vi "Fast Pixel to Micron.vi"(0 "Refnum In":T2, 11 "error in (no error)":errorcluster, 12 "Conversion Method":u16(ring)=1 items=["Strip Centers", "Signal Fit, Left to Right", "Projection + Signal Fit"]) -> (3 "FFT Angle (Rad)":dbl format="%_6f", 4 "Microns/Pixel":dbl format="%.4f", 6 "Error":dbl format="%.4f", 8 "Corrected":dbl format="%.4f", 10 "Error":dbl format="%.4f", 14 "FFT Error (Rad)":dbl format="%_6f", 15 "error out":errorcluster)   [LabVIEW 2016]
uses:
  <vilib>/Analysis/6fits.llb/Curve Fitting Criteria.ctl
  <vilib>/vision/Image Controls.llb/IMAQ Image.ctl
  <vilib>/measure/mascope.llb/Pulse Measurements 1 chan.vi
  <vilib>/measure/matone.llb/Extract Single Tone Information 1 Chan.vi
  <vilib>/vision/NI_Vision_Development_Module.lvlib
  <vilib>/Analysis/NI_AALBase.lvlib
  <vilib>/measure/NI_MAPro.lvlib
  <vilib>/Analysis/NI_AALPro.lvlib
  <vilib>/Analysis/6fits.llb/Remove Outliers (Range).vi
  <vilib>/Analysis/6fits.llb/Confidence Interval (Linear).vi
panel:
  in  "Tab Control":T1(tab)
  out "Original Image":T2(plugin-control)
  in  "File Path":path=path "D:/Documents/School/Brookhaven/Images/2017-06-15/image_004_600_60_15.png"
  out "Cropped Image":T2(plugin-control)
  in  "Crop Size":i32=1000 min=250 max=2700
  out "Thresholded Image":T2(plugin-control)
  out "FFT Skew Detection":T2(plugin-control)
  in  "Fit Method":T3 items=["Least Square", "Least Absolute Residual", "Bisquare"]
  out "Fit Slopes":dbl[](array[numeric]) format="%^_3e"
  out "Error (Slope)":dbl format="%.5f"
  out "Error (Radians)":dbl format="%.5f"
  out "Radians":dbl format="%.5f"
  out "Slope":dbl format="%.5f"
  in  "Minimum Width":i32=7 min=3 max=15
  in  "Point Constraint (Pixels)":dbl=40.0 min=0.0 max=100.0 step=1.0 format="%#.2f"
  in  "Keep N Devs":dbl=2.0 min=1.0 max=5.0
  in  "Minimum Height":dbl=200.0 min=0.0 max=255.0
  out "Num slope errors":i32
  out "Num slopes":i32
  in  "Use Center Nth of Strips":i32=4 min=1 max=10 step=1
  out "Slope Error":dbl[](array[numeric]) format="%^#_3e"
  out "FFT Angle (Deg)":dbl format="%_6g"
  out "FFT Error (Deg)":dbl format="%_6g"
  out "Distribution of Pitches":T4(graph)
  out "Mean (Pixels)":dbl format="%.4f"
  out "Std. Dev.":dbl format="%.4f"
  out "N":i32
  out "Std. Dev / Sqrt(N)":dbl format="%#.4g"
  in  "Max Value":dbl=70.0 format="%#_13g"
  in  "Min Value":dbl=40.0 min=30.0 max=75.0
  in  "Standard Devs":dbl=3.0 min=0.0 max=5.0
  # "FFT Skew Detection"
  # "Pixel to Micron Conversion"
  # "Histogram"
  # "Absolute Constraint"
  # "Relative Constraint"
  # "Skew Correction (Experimental)"
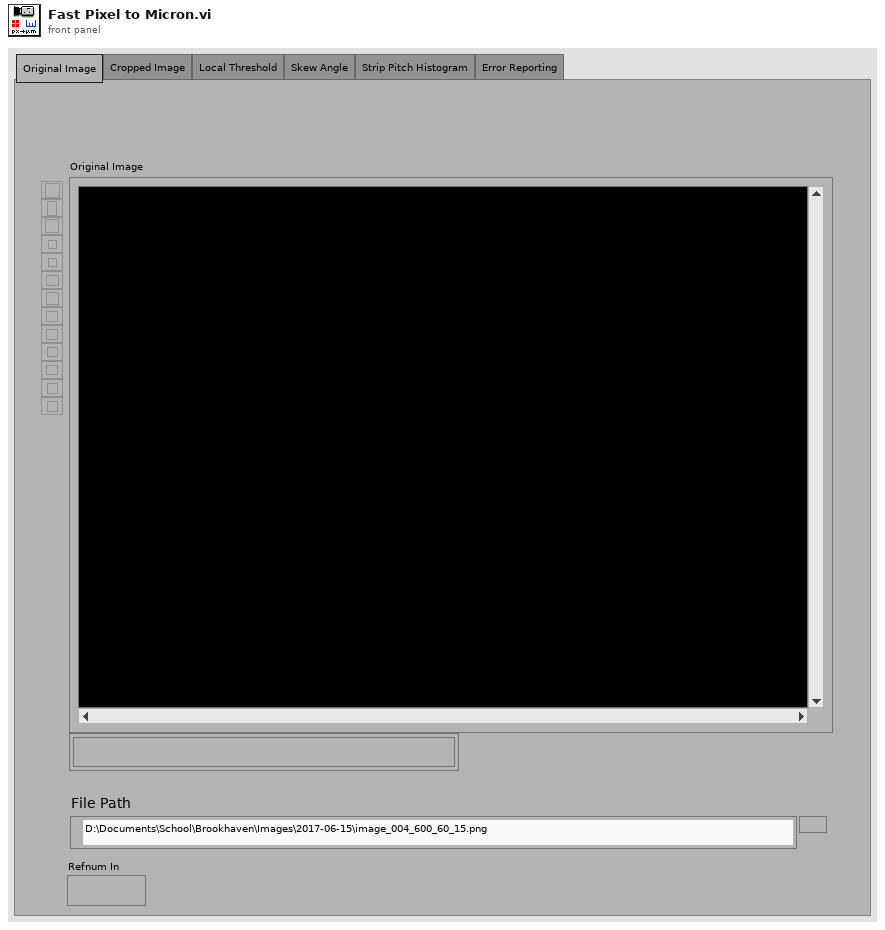
[diagram p1: front panel]
types:
  T1 = enum32{"Original Image", "Cropped Image", "Local Threshold", "Skew Angle", "Strip Pitch Histogram", "Error Reporting"}
  T2 = typedef "IMAQ Image.ctl" = refnum<image>
  T3 = typedef "NI_AALPro.lvlib/Curve Fitting Criteria.ctl" = u16
  T4 = cluster{"X Values":dbl[], "Histogram: h(x)":i32[]}
  T5 = typedef "Image Type" = u32
  T6 = cluster{"high ref level":dbl, "mid ref level":dbl, "low ref level":dbl, "ref units":u16}
  T7 = cluster{"pulse center":dbl, "ref levels":cluster{"high ref level":dbl, "mid ref level":dbl, "low ref level":dbl, "ref units":u16}}
  T8 = cluster{"Numeric":dbl, "Numeric":dbl, "Numeric":dbl}[]
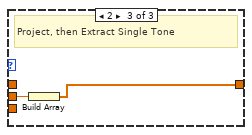
[diagram p10: hidden frame]
diagram:
  n1 = Not A Number/Path/Refnum?(number/path/refnum="Refnum In") -> (NaN/Path/Refnum?=w4:bool)
  n2 = case shown="True" w4 {
    tunnel: [w49 w52] -> w47
    tunnel: [w48 w51] -> w20
    tunnel: "error in (no error)" -> [w48 w50]
    tunnel: "Refnum In" -> [w49 _]
    frame False {
    }
    frame True {
      n3 = in-place {
        in-place-border: [w58] -> w52
        in-place-border: [w55] -> w51
        in-place-border: w50 -> [w54]
        w59 = T5 0 items=["Grayscale (U8)", "Grayscale (I16)", "Grayscale (SGL)", "Complex (CSG)", "RGB (U32)", "HSL (U32)", "RGB (U64)", "Grayscale (U16)"] ("Image Type")
        # "Load test image"
        n4 = call "IMAQ Create"("Image Name"="Test Image", "Image Type"=w59, "error in (no error)"=w54) -> ("New Image"=w60:T2, "error out"=w56:errorcluster)  [unwired: 2 in]
        n5 = call "IMAQ ReadFile"("File Path"="File Path", "error in (no error)"=w56, "Load Color Palette? (No)"=FALSE, "Image"=w60) -> ("error out"=w55:errorcluster, "Image Out"=w58:T2)  [unwired: 3 in, 3 out]
      }
    }
  }
  "Original Image" <- w47
  n6 = in-place {
    in-place-border: [w83] -> w2
    in-place-border: w47 -> [w71]
    in-place-border: w20 -> [w65]
    in-place-border: [w62] -> w1
    w70 = 2.0
    w82 = T5 0 items=["Grayscale (U8)", "Grayscale (I16)", "Grayscale (SGL)", "Complex (CSG)", "RGB (U32)", "HSL (U32)", "RGB (U64)", "Grayscale (U16)"] ("Image Type")
    # "Crop region of interest"
    n7 = call "IMAQ GetImageSize"("Image"=w71, "error in (no error)"=w65) -> ("Y Resolution"=w79:i32, "X Resolution"=w81:i32, "error out"=w64:errorcluster)  [unwired: 2 in]
    n8 = Subtract(x=w81, y="Crop Size") -> (x-y=w68:i32)
    n9 = Subtract(x=w79, y="Crop Size") -> (x-y=w66:i32)
    n10 = To Double Precision Float(number=w68) -> (double precision float=w69:dbl)
    n11 = To Double Precision Float(number=w66) -> (double precision float=w67:dbl)
    n12 = Divide(x=w69, y=w70) -> (x/y=w80:dbl)
    n13 = Divide(x=w67, y=w70) -> (x/y=w78:dbl)
    n14 = To Unsigned Long Integer(number=w80) -> (unsigned 32bit integer=w77:u32)
    n15 = To Unsigned Long Integer(number=w78) -> (unsigned 32bit integer=w75:u32)
    n16 = Add(x=w77, y="Crop Size") -> (x+y=w76:u32)
    n17 = Add(x=w75, y="Crop Size") -> (x+y=w73:u32)
    n18 = call "IMAQ Create"("Image Name"="Crop", "Image Type"=w82, "error in (no error)"=w64) -> ("New Image"=w84:T2, "error out"=w63:errorcluster)  [unwired: 2 in]
    n19 = Build Array(w77, w75, w76, w73) -> (w72:u32[])
    n20 = call "IMAQ Extract 2"("Optional Rectangle"=w72, "error in (no error)"=w63, "Image Dst"=w84, "Image Src"=w71) -> ("error out"=w62:errorcluster, "Image Dst Out"=w83:T2)  [unwired: 6 in]
  }
  "Cropped Image" <- w2
  n21 = in-place {
    in-place-border: w2 -> [w97]
    in-place-border: [w90] -> w12
    in-place-border: w1 -> [w89]
    in-place-border: [w87] -> w11
    w91 = T5 0 items=["Grayscale (U8)", "Grayscale (I16)", "Grayscale (SGL)", "Complex (CSG)", "RGB (U32)", "HSL (U32)", "RGB (U64)", "Grayscale (U16)"] ("Image Type")
    w95 = u32 0 items=["Niblack", "Background Correction", "Sauvola"] ("Method (Niblack)")
    w96 = u32 0 items=["Bright Objects", "Dark Objects"] ("Look For (Bright Objects)")
    # "Apply adaptive threshold"
    n22 = call "IMAQ Create"("Image Name"="Threshold", "Image Type"=w91, "error in (no error)"=w89) -> ("New Image"=w93:T2, "error out"=w88:errorcluster)  [unwired: 2 in]
    n23 = call "IMAQ Local Threshold"("Image Src"=w97, "Look For (Bright Objects)"=w96, "Method (Niblack)"=w95, "Image Dst"=w93, "Window Size (32x32)"=cluster{"SizeX":i32, "SizeY":i32} {"SizeX"=101, "SizeY"=101}, "error in (no error)"=w88, "Niblack/Sauvola Deviation Factor (0.2)"=0.15, "Replace Value (1)"=sgl 255.0) -> ("Image Dst Out"=w90:T2, "error out"=w87:errorcluster)  [unwired: 6 in]
  }
  "Thresholded Image" <- w12
  n24 = in-place {
    in-place-border: w12 -> [w105]
    in-place-border: [w102] -> w44
    in-place-border: w11 -> [w101]
    in-place-border: [w99] -> w10
    # "Sample image from left to right, collect period of each signal"
    n25 = call "IMAQ GetImageSize"("Image"=w105, "error in (no error)"=w101) -> ("Y Resolution"=w103:i32, "X Resolution"=w104:i32, "error out"=w100:errorcluster)  [unwired: 2 in]
    n26 = for {
      N: w104 -> [_]
      tunnel: w105 -> [w117]
      tunnel: w103 -> [w114]
      tunnel: [w109] -> w102 mode=indexing
      tunnel: w100 -> [w108]
      tunnel: [w106] -> w99 mode=indexing
      i -> [w116]
      n27 = Build Array "Create Line"(w116, 0 ("element"), w116, w114) -> (w112:i32[])
      n28 = call "IMAQ LineProfile"("error in (no error)"=w108, "Line Coordinates"=w112, "Image"=w117) -> ("error out"=w107:errorcluster, "Line Graph"=w113:cluster{"x0":sgl, "dx":sgl, "Pixels Line":sgl[]})  [unwired: 2 in, 2 out]
      n29 = Unbundle(w113) -> ("Pixels Line"=w111:sgl[])  [unwired: 2 out]
      n30 = call-poly <vilib>:"Extract Single Tone Information.vi"("error in (no error)"=w107, "time signal in"=w111) -> ("error out"=w106:errorcluster, "detected frequency"=w110:dbl)  [unwired: 4 in, 4 out]
      n31 = Reciprocal(x=w110) -> (1/x=w109:dbl)
    }
  }
  n32 = in-place {
    in-place-border: w12 -> [w124]
    in-place-border: [w121] -> w41
    in-place-border: w11 -> [w120]
    in-place-border: [w118] -> w19
    # "Project, then get period of signal"
    n33 = call "IMAQ LinearAverages"("error in (no error)"=w120, "Image Src"=w124) -> ("error out"=w119:errorcluster, "Y Axis Averages"=w123:sgl[])  [unwired: 5 in, 3 out]
    n34 = call-poly <vilib>:"Extract Single Tone Information.vi"("error in (no error)"=w119, "time signal in"=w123) -> ("error out"=w118:errorcluster, "detected frequency"=w122:dbl)  [unwired: 4 in, 4 out]
    n35 = Reciprocal(x=w122) -> (1/x=w121:dbl)
  }
  n36 = call "FFT Skew Detection.vi"("error in (no error)"=w11, "Refnum In"=w12) -> ("error out"=w9:errorcluster, "Error (Degrees)"=→"FFT Error (Deg)":dbl, "Error (Radians)"=w13:dbl, "Fit Line"=→"FFT Skew Detection":T2, "Alt. Angle (Degrees)"=→"FFT Angle (Deg)":dbl, "Alt. Angle (Radians)"=w8:dbl)  [unwired: 2 in, 2 out]
  "FFT Angle (Rad)" <- w8
  "FFT Error (Rad)" <- w13
  n37 = call "IMAQ GetImageSize"("Image"=w12, "error in (no error)"=w11) -> ("Y Resolution"=w46:i32, "X Resolution"=w32:i32, "error out"=w18:errorcluster)  [unwired: 2 in]
  n38 = To Double Precision Float(number=w32) -> ()  [unwired: 1 out]
  n39 = for {
    N: w32 -> [_]
    tunnel: w12 -> [w128]
    tunnel: w46 -> [w142]
    tunnel: [w141] -> _ mode=concatenating
    tunnel: [w139] -> w26 mode=concatenating
    tunnel: [w137] -> w29 mode=concatenating
    tunnel: [w132] -> w28 mode=concatenating
    tunnel: [w129] -> w43 mode=concatenating
    tunnel: w18 -> [w127]
    tunnel: [w125] -> w17 mode=concatenating
    i -> [w140]
    # "List of strip centers"
    n40 = Build Array "Create Line"(w140, 0 ("element"), w140, w142) -> (w144:i32[])
    n41 = call "IMAQ LineProfile"("error in (no error)"=w127, "Line Coordinates"=w144, "Image"=w128) -> ("error out"=w126:errorcluster, "Line Graph"=w143:cluster{"x0":sgl, "dx":sgl, "Pixels Line":sgl[]})  [unwired: 2 in, 2 out]
    n42 = in-place {
      in-place-border: w143 -> [w151]
      in-place-border: [w148] -> w138
      in-place-border: [w147] -> w136
      in-place-border: [w146] -> w135
      # "Get list of peaks matching a threshold and width"
      n43 = Unbundle(w151) -> ("Pixels Line"=w148:sgl[])  [unwired: 2 out]
      n44 = call <vilib>:"Threshold Detector.vi"("width"="Minimum Width", "threshold"="Minimum Height", "X"=w148) -> ("count"=w146:i32, "Indices"=w147:i32[])  [unwired: 1 out]
    }
    n45 = Subtract(x=w135, y=2) -> (x-y=w131:i32)
    n46 = for {
      N: w131 -> [_]
      tunnel: w138 -> [w172]
      tunnel: [w166] -> w130 mode=indexing
      tunnel: w136 -> [w169]
      tunnel: [w161] -> w133 mode=indexing
      tunnel: w126 -> [w160]
      tunnel: [w159] -> w125 mode=indexing
      i -> [w165]
      w174 = u16 0 items=["all", "no period and duty cycle"] ("export mode")
      w175 = u16 1 items=["low pulse", "high pulse"] ("polarity (high)")
      # "Iterate list of peak indices, analyzing each pulse"
      n47 = Increment(x=w165) -> (x+1=w164:i32)
      n48 = Index Array(array=w169, index=w164) -> (element=w167:i32)
      n49 = Decrement(x=w167) -> (x-1=w168:i32)
      n50 = Array Subset(array=w172, index=w168) -> (w171:sgl[])  [unwired: 1 in]
      n51 = call-poly <vilib>:"Pulse Measurements.vi"("export mode"=w174, "pulse number (1)"=1, "error in (no error)"=w160, "reference levels"=T6 {"high ref level"=210.0, "mid ref level"=100.0, "low ref level"=10.0, "ref units"=0}, "polarity (high)"=w175, "signal in"=w171) -> ("error out"=w159:errorcluster, "pulse duration"=w162:dbl, "measurement info"=w173:T7)  [unwired: 1 in, 2 out]
      n52 = in-place {
        in-place-border: w162 -> [w181]
        in-place-border: [w180] -> w161
        # "Estimate errors on strip centers"
        n53 = Square(x=w181) -> (x^2=w186:dbl)
        n54 = Divide(x=1.0, y=3.0) -> (x/y=w187:dbl)
        n55 = Multiply(x=w187, y=w186) -> (x*y=w185:dbl)
        n56 = Square Root(x=w185) -> (sqrt(x)=w184:dbl)
        n57 = Divide(x=w184, y=2.0) -> (x/y=w182:dbl)
        n58 = Divide(x=w182, y=w181) -> (x/y=w180:dbl)
      }
      n59 = in-place {
        in-place-border: w173 -> [w179]
        in-place-border: w167 -> [w177]
        in-place-border: [w176] -> w166
        # "Calculate strip centers"
        n60 = Unbundle(w179) -> ("pulse center"=w178:dbl)  [unwired: 1 out]
        n61 = Add(x=w178, y=w177) -> (x+y=w176:dbl)
      }
    }
    n62 = in-place {
      in-place-border: w130 -> [w157]
      in-place-border: [w154] -> w129
      w158 = u16 2 items=["2nd Order Central", "4th Order Central", "Forward", "Backward"] ("method")
      # "Calculate inter-strip distances"
      n63 = call <vilib>:"Derivative x(t).vi"("method"=w158, "X"=w157) -> ("dX/dt"=w156:dbl[])  [unwired: 8 in, 1 out]
      n64 = Array Size(array=w156) -> (size(s)=w155:i32)
      n65 = Decrement(x=w155) -> (x-1=w152:i32)
      n66 = Array Subset(array=w156, index=0, length=w152) -> (w154:dbl[])
    }
    n67 = Build Array(w140) -> (w139:i32[])
    n68 = Build Array(w136) -> (w141:i32[][])
    n69 = Build Array(w133) -> (w132:dbl[][])
    n70 = Build Array(w130) -> (w137:dbl[][])
  }
  n71 = disable-structure shown="Disabled" {
    disable-tunnel: w29 -> [w194 _]
    disable-tunnel: w28 -> [w193 _]
    disable-tunnel: "Point Constraint (Pixels)" -> [w192 _]
    disable-tunnel: w26 -> [w191 _]
    disable-tunnel: [w190 _] -> w25
    frame Disabled {
      n72 = in-place {
        in-place-border: w194 -> [w207]
        in-place-border: w193 -> [w196]
        in-place-border: w192 -> [w199]
        in-place-border: w191 -> [w201]
        in-place-border: [w198] -> w190
        # "Realign shifted array values due to dirt/skew"
        n73 = Transpose 2D Array(2D array=w196) -> (transposed array=w197:dbl[][])
        n74 = Transpose 2D Array(2D array=w207) -> (transposed array=w202:dbl[][])
        n75 = in-place {
          in-place-border: [w211] -> w195
          in-place-border: [w210] -> _
          in-place-border: w197 -> [w208]
          # "Create 1D array of Weights"
          n76 = Array Size(array=w208) -> (size(s)=w210:i32[])
          n77 = Multiply Array Elements(1:w210) -> (0:w209:i32)
          n78 = Reshape Array(w208, w209) -> (w211:dbl[])
        }
        n79 = in-place {
          in-place-border: [w215] -> w206
          in-place-border: [w214] -> w204
          in-place-border: w202 -> [w212]
          # "Create 1D array of Y values"
          n80 = Array Size(array=w212) -> (size(s)=w214:i32[])
          n81 = Multiply Array Elements(1:w214) -> (0:w213:i32)
          n82 = Reshape Array(w212, w213) -> (w215:dbl[])
        }
        n83 = Index Array(array=w204, index=0) -> (element=w203:i32)
        n84 = for {
          N: w203 -> [_]
          tunnel: w201 -> [w216]
          tunnel: [w216] -> w200 mode=concatenating
          # "Create 1D array of X values, repeated for each strip"
        }
        n85 = for {
          tunnel: w202 -> [w234] mode=indexing
          tunnel: w206 -> [w226]
          tunnel: w200 -> [w231]
          tunnel: w199 -> [w233]
          tunnel: [w224] -> w198 mode=indexing
          tunnel: w195 -> [w223]
          w232 = u16 0 items=["Y", "X", "X and Y"] ("range type")
          # "Using the median of each row, collect all strip centers (X,Y) within a constrained distance from the median"
          n86 = call <vilib>:"Median.vi"("X"=w234) -> ("median"=w228:dbl)  [unwired: 1 out]
          n87 = Add(x=w228, y=w233) -> (x+y=w230:dbl)
          n88 = Subtract(x=w228, y=w233) -> (x-y=w229:dbl)
          n89 = To Double Precision Float(number=w231) -> (double precision float=w225:dbl[])
          n90 = Build Array(w230, w229) -> (w227:dbl[])
          n91 = call-poly <vilib>:"Remove Outliers.vi"("Y"=w226, "X"=w225, "Weight"=w223, "range type"=w232, "Range"=w227) -> ("Y Out"=w221:dbl[], "X Out"=w222:dbl[], "Weight Out"=w220:dbl[])  [unwired: 6 in, 2 out]
          n92 = in-place {
            in-place-border: w222 -> [w242]
            in-place-border: w221 -> [w241]
            in-place-border: w220 -> [w240]
            in-place-border: [w237] -> w219
            in-place-border: [w236] -> w218
            in-place-border: [w235] -> w217
            # "Sort by X value"
            n93 = Build Cluster Array(w242, w241, w240) -> (w239:T8)
            n94 = Sort 1D Array(array=w239) -> (sorted array=w238:T8)
            n95 = for {
              tunnel: w238 -> [w246] mode=indexing
              tunnel: [w244] -> _ mode=indexing
              tunnel: [w243] -> _ mode=indexing
              tunnel: [w245] -> _ mode=indexing
              tunnel: [w245] -> w237 mode=indexing
              tunnel: [w244] -> w236 mode=indexing
              tunnel: [w243] -> w235 mode=indexing
              n96 = Unbundle(w246) -> ("Numeric"=w244:dbl, "Numeric"=w243:dbl, "Numeric"=w245:dbl)
            }
          }
          n97 = Bundle(w217, w218, w219) -> (w224:cluster{dbl[], dbl[], dbl[]})  [unwired: 1 in]
        }
      }
    }
    frame Enabled {
    }
  }
  n98 = Merge Errors(w9, w10, w19, w17) -> (w16:errorcluster)
  n99 = case shown="1, Default" "Conversion Method" {
    tunnel: w44 -> [_ w248 _]
    tunnel: [w247 w248 w249] -> w40
    tunnel: w43 -> [w247 _ _]
    tunnel: w41 -> [_ _ w250]
    frame 0 {
      # "Distance between strip centers"
    }
    frame 1, Default {
      # "Line Profile, then Extract Single Tone"
    }
    frame 2 {
      # "Project, then Extract Single Tone"
      n100 = Build Array(w250) -> (w249:dbl[])
    }
  }
  n101 = Array Size(array=w40) -> (size(s)=w39:i32)
  n102 = Greater?(x=w39, y=1) -> (0:w37:bool)
  n103 = case shown="True" w37 {
    tunnel: w40 -> [w251 w253]
    tunnel: [w251 w252] -> w36
    frame False {
      # "Array is a single value, so do nothing"
    }
    frame True {
      # "If the array has more than one element, perform histogram constaints"
      n104 = in-place {
        in-place-border: [w264] -> w254
        in-place-border: w253 -> [w263]
        # "Absolute constraint on values"
        n105 = In Range and Coerce(upper limit="Max Value", x=w263, lower limit="Min Value") -> (coerced(x)=w264:dbl[])  [unwired: 1 out]
      }
      n106 = in-place {
        in-place-border: w254 -> [w256]
        in-place-border: [w255] -> w252
        # "Constrain to n Standard Deviations"
        n107 = call <vilib>:"Std Deviation and Variance.vi"("X"=w256) -> ("mean"=w259:dbl, "standard deviation"=w261:dbl)  [unwired: 1 in, 1 out]
        n108 = Multiply(x="Standard Devs", y=w261) -> (x*y=w258:dbl)
        n109 = Add(x=w258, y=w259) -> (x+y=w260:dbl)
        n110 = Subtract(x=w259, y=w258) -> (x-y=w257:dbl)
        n111 = In Range and Coerce(upper limit=w260, x=w256, lower limit=w257) -> (coerced(x)=w255:dbl[])  [unwired: 1 out]
      }
    }
  }
  n112 = in-place {
    in-place-border: [w269] -> w34
    in-place-border: [w267] -> _
    in-place-border: [w268] -> w35
    in-place-border: w36 -> [w267]
    # "Histogram"
    n113 = call <vilib>:"Std Deviation and Variance.vi"("X"=w267) -> ("mean"=w268:dbl, "standard deviation"=w269:dbl)  [unwired: 1 in, 1 out]
    "Mean (Pixels)" <- w268
    "Std. Dev." <- w269
    n114 = call <vilib>:"Histogram.vi"("X"=w267) -> ("Histogram Graph"=→"Distribution of Pitches":T4)  [unwired: 7 in, 3 out]
  }
  n115 = in-place {
    in-place-border: w34 -> [w274]
    in-place-border: w35 -> [w278]
    in-place-border: [w273] -> w33
    in-place-border: w40 -> [w275]
    in-place-border: [w272] -> w21
    in-place-border: w16 -> [w271]
    in-place-border: [w271] -> w14
    # "Pixel to Micron Conversion with Error"
    n116 = Array Size(array=w275) -> (size(s)=w277:i32)
    "N" <- w277
    n117 = To Double Precision Float(number=w277) -> (double precision float=w276:dbl)
    n118 = Divide(x=74.5, y=w278) -> (x/y=w273:dbl)
    "Microns/Pixel" <- w273
    n119 = Square(x=w273) -> (x^2=w280:dbl)
    n120 = Square Root(x=w276) -> (sqrt(x)=w282:dbl)
    n121 = Reciprocal(x=w280) -> (1/x=w279:dbl)
    n122 = Divide(x=w274, y=w282) -> (x/y=w281:dbl)
    "Std. Dev / Sqrt(N)" <- w281
    n123 = Multiply(x=w279, y=w281) -> (x*y=w272:dbl)
    "Error" <- w272
  }
  "error out" <- w14
  n124 = disable-structure shown="Disabled" {
    disable-tunnel: w29 -> [w290 _]
    disable-tunnel: w28 -> [w289 _]
    disable-tunnel: w26 -> [w288 _]
    disable-tunnel: w25 -> [w287 _]
    disable-tunnel: [w286 _] -> w24
    disable-tunnel: [w285 _] -> w23
    disable-tunnel: [w284 _] -> w22
    frame Disabled {
      n125 = in-place {
        in-place-border: w290 -> [w301]
        in-place-border: [w301] -> _
        in-place-border: w288 -> [w296]
        in-place-border: [w296] -> _
        in-place-border: w289 -> [w300]
        in-place-border: [w300] -> w291
        in-place-border: w287 -> [w298]
        in-place-border: [w294] -> w286
        in-place-border: [w293] -> w285
        in-place-border: [w292] -> w284
        # "Take only the middle Nth of strips"
        n126 = Array Size(array=w298) -> (size(s)=w299:i32)
        n127 = in-place {
          in-place-border: "Use Center Nth of Strips" -> [w336]
          in-place-border: w299 -> [w330]
          in-place-border: w298 -> [w328]
          in-place-border: [w324] -> w297
          # "Subset of the center strips"
          n128 = To Double Precision Float(number=w330) -> (double precision float=w329:dbl)
          n129 = Divide(x=w329, y=w336) -> (x/y=w331:dbl)
          n130 = Divide(x=w329, y=2.0) -> (x/y=w334:dbl)
          n131 = Round To Nearest(number=w331) -> (nearest integer value=w326:dbl)
          n132 = Divide(x=w326, y=2.0) -> (x/y=w333:dbl)
          n133 = Subtract(x=w334, y=w333) -> (x-y=w332:dbl)
          n134 = To Long Integer(number=w332) -> (32bit integer=w327:i32)
          n135 = To Long Integer(number=w326) -> (32bit integer=w325:i32)
          n136 = Array Subset(array=w328, index=w327, length=w325) -> (w324:cluster{dbl[], dbl[], dbl[]}[])
        }
        n137 = for {
          tunnel: w297 -> [w323] mode=indexing
          tunnel: w296 -> [w322]
          tunnel: "Use Center Nth of Strips" -> [w314]
          tunnel: [w304] -> w294 mode=indexing
          tunnel: [w303] -> w293 mode=indexing
          tunnel: [w302] -> w292 mode=indexing
          w308 = u16 1 items=["Y", "X", "X and Y"] ("range type")
          n138 = Array Size(array=w322) -> (size(s)=w313:i32)
          n139 = To Double Precision Float(number=w313) -> (double precision float=w316:dbl)
          n140 = Divide(x=w316, y=w314) -> (x/y=w317:dbl)
          n141 = Divide(x=w316, y=2.0) -> (x/y=w319:dbl)
          n142 = Round To Nearest(number=w317) -> (nearest integer value=w315:dbl)
          n143 = Divide(x=w315, y=2.0) -> (x/y=w318:dbl)
          n144 = Subtract(x=w319, y=w318) -> (x-y=w306:dbl)
          n145 = To Long Integer(number=w315) -> (32bit integer=w312:i32)
          n146 = To Long Integer(number=w306) -> ()  [unwired: 1 out]
          n147 = Add(x=w306, y=w312) -> (x+y=w307:dbl)
          n148 = Build Array(w307, w306) -> (w305:dbl[])
          n149 = Unbundle(w323) -> (w311:dbl[], w310:dbl[], w309:dbl[])
          n150 = call-poly <vilib>:"Remove Outliers.vi"("Y"=w311, "X"=w310, "Weight"=w309, "range type"=w308, "Range"=w305) -> ("Y Out"=w303:dbl[], "X Out"=w304:dbl[], "Weight Out"=w302:dbl[])  [unwired: 6 in, 2 out]
        }
      }
      n151 = Transpose 2D Array(2D array=w291) -> ()  [unwired: 1 out]
    }
    frame Enabled {
    }
  }
  n152 = in-place {
    in-place-border: w8 -> [w338]
    in-place-border: w33 -> [w341]
    in-place-border: w13 -> [w340]
    in-place-border: w21 -> [w339]
    # "Correction"
    n153 = in-place {
      in-place-border: w341 -> [w352]
      in-place-border: w338 -> [w354]
      in-place-border: w340 -> [w349]
      in-place-border: w339 -> [w357]
      # "Calculate error on the correction"
      n154 = Secant(1:w354) -> (0:w355:dbl)
      n155 = Tangent(1:w354) -> (0:w353:dbl)
      n156 = Cosine(x=w354) -> (cos(x)=w359:dbl)
      n157 = Multiply(x=w355, y=w353) -> (x*y=w351:dbl)
      n158 = Reciprocal(x=w359) -> (1/x=w358:dbl)
      n159 = Multiply(x=w351, y=w352) -> (x*y=w350:dbl)
      n160 = Multiply(x=w358, y=w357) -> (x*y=w356:dbl)
      n161 = Multiply(x=w350, y=w349) -> (x*y=w348:dbl)
      n162 = Square(x=w356) -> (x^2=w346:dbl)
      n163 = Square(x=w348) -> (x^2=w347:dbl)
      n164 = Add(x=w347, y=w346) -> (x+y=w345:dbl)
      n165 = Square Root(x=w345) -> (sqrt(x)=→"Error":dbl)
    }
    n166 = Cosine(x=w338) -> (cos(x)=w343:dbl)
    n167 = Divide(x=w341, y=w343) -> (x/y=→"Corrected":dbl)
  }
  n168 = disable-structure shown="Disabled" {
    disable-tunnel: [w366 _] -> w45
    disable-tunnel: [w365 _] -> w31
    disable-tunnel: [w364 _] -> w30
    disable-tunnel: "Point Constraint (Pixels)" -> [w363 _]
    disable-tunnel: w24 -> [w362 _]
    disable-tunnel: w23 -> [w361 _]
    disable-tunnel: w22 -> [w360 _]
    frame Disabled {
      n169 = for {
        tunnel: w361 -> [w367] mode=indexing
        tunnel: [w371] -> w366 mode=indexing
        tunnel: [w379] -> _ mode=indexing
        tunnel: w360 -> [w375] mode=indexing
        tunnel: [w376] -> w365 mode=indexing
        tunnel: [w370] -> w364 mode=indexing
        tunnel: w363 -> [w369]
        tunnel: w362 -> [w368] mode=indexing
        # "Exclude outliers, fit strip centers with estimated weights"
        n170 = in-place {
          in-place-border: w375 -> [w392]
          in-place-border: [w391] -> w374
          in-place-border: [w390] -> w373
          in-place-border: [w389] -> w372
          in-place-border: w369 -> [w387]
          in-place-border: w368 -> [w386]
          in-place-border: w367 -> [w384]
          w399 = u16 0 items=["Y", "X", "X and Y"] ("range type")
          # "Exclude outliers"
          n171 = call <vilib>:"Std Deviation and Variance.vi"("X"=w384) -> ()  [unwired: 1 in, 3 out]
          n172 = Square Root(x=w392) -> (sqrt(x)=w394:dbl[])
          n173 = call <vilib>:"Median.vi"("X"=w384) -> ("median"=w385:dbl)  [unwired: 1 out]
          n174 = Multiply(x=w387, y=1.0) -> (x*y=w398:dbl)
          n175 = Add(x=w385, y=w398) -> (x+y=w396:dbl)
          n176 = Subtract(x=w385, y=w398) -> (x-y=w395:dbl)
          n177 = Reciprocal(x=w394) -> (1/x=w393:dbl[])
          n178 = Build Array(w396, w395) -> (w397:dbl[])
          n179 = call-poly <vilib>:"Remove Outliers.vi"("Y"=w384, "X"=w386, "Weight"=w393, "range type"=w399, "Range"=w397) -> ("Y Out"=w391:dbl[], "X Out"=w390:dbl[], "Weight Out"=w389:dbl[])  [unwired: 6 in, 2 out]
        }
        n180 = in-place {
          in-place-border: w374 -> [w422]
          in-place-border: [w420] -> w378
          w418 = 0 ("index")
          w425 = u16 2 items=["2nd Order Central", "4th Order Central", "Forward", "Backward"] ("method")
          # "dY"
          n181 = call <vilib>:"Derivative x(t).vi"("method"=w425, "X"=w422) -> ("dX/dt"=w424:dbl[])  [unwired: 8 in, 1 out]
          n182 = Array Size(array=w424) -> (size(s)=w423:i32)
          n183 = Decrement(x=w423) -> (x-1=w419:i32)
          n184 = Subtract(x=w419, y=w418) -> (x-y=w417:i32)
          n185 = Array Subset(array=w424, index=w418, length=w417) -> (w421:dbl[])
          n186 = Negate(x=w421) -> (-x=w420:dbl[])
        }
        n187 = in-place {
          in-place-border: w373 -> [w413]
          in-place-border: [w412] -> w377
          w410 = 0 ("index")
          w416 = u16 2 items=["2nd Order Central", "4th Order Central", "Forward", "Backward"] ("method")
          # "dX"
          n188 = call <vilib>:"Derivative x(t).vi"("method"=w416, "X"=w413) -> ("dX/dt"=w415:dbl[])  [unwired: 8 in, 1 out]
          n189 = Array Size(array=w415) -> (size(s)=w414:i32)
          n190 = Decrement(x=w414) -> (x-1=w411:i32)
          n191 = Subtract(x=w411, y=w410) -> (x-y=w409:i32)
          n192 = Array Subset(array=w415, index=w410, length=w409) -> (w412:dbl[])
        }
        n193 = in-place {
          in-place-border: w374 -> [w406]
          in-place-border: w373 -> [w405]
          in-place-border: w372 -> [w404]
          in-place-border: [w403] -> w371
          in-place-border: [w400] -> w370
          # "Linear fit to strips, with fit error"
          n194 = call <vilib>:"Linear Fit.vi"("Y"=w406, "X"=w405, "Weight"=w404, "tolerance"=1e-06, "method"="Fit Method") -> ("slope"=w403:dbl, "intercept"=w402:dbl)  [unwired: 6 in, 3 out]
          n195 = call-poly <vilib>:"Linear Fit Intervals.vi"("Y"=w406, "confidence level"=0.68, "X"=w405, "Weight"=w404, "slope"=w403, "intercept"=w402) -> ("delta slope"=w400:dbl)  [unwired: 5 in, 4 out]
        }
        n196 = Bundle("X Out"=w373, "Y Out"=w374) -> (w379:cluster{"X Out":dbl[], "Y Out":dbl[]})  [unwired: 1 in]
        n197 = in-place {
          in-place-border: w378 -> [w383]
          in-place-border: w377 -> [w382]
          in-place-border: [w380] -> w376
          # "Collect angles"
          n198 = Divide(x=w383, y=w382) -> (x/y=w381:dbl[])
          n199 = Inverse Tangent(1:w381) -> (0:w380:dbl[])
        }
      }
    }
    frame Enabled {
    }
  }
  n200 = disable-structure shown="Disabled" {
    disable-tunnel: w31 -> [w426 _]
    frame Disabled {
      n201 = in-place {
        in-place-border: [w432] -> w427
        in-place-border: w426 -> [w431]
        # "Reshape into 1D array"
        n202 = Array Size(array=w431) -> (size(s)=w430:i32[])
        n203 = Multiply Array Elements(1:w430) -> (0:w429:i32)
        n204 = Reshape Array(w431, w429) -> (w432:dbl[])
      }
      n205 = in-place {
        in-place-border: w427 -> [w437]
        in-place-border: [w436] -> w428
        # "Constrain angles to n Standard Deviations"
        n206 = call <vilib>:"Std Deviation and Variance.vi"("X"=w437) -> ("mean"=w440:dbl, "standard deviation"=w442:dbl)  [unwired: 1 in, 1 out]
        n207 = Multiply(x=3.0 ("Angle Constraint (Std. Devs)"), y=w442) -> (x*y=w439:dbl)
        n208 = Add(x=w439, y=w440) -> (x+y=w441:dbl)
        n209 = Subtract(x=w440, y=w439) -> (x-y=w438:dbl)
        n210 = In Range and Coerce(upper limit=w441, x=w437, lower limit=w438) -> (coerced(x)=w436:dbl[])  [unwired: 1 out]
      }
      n211 = in-place {
        in-place-border: [w435] -> _
        in-place-border: [w434] -> _
        in-place-border: w428 -> [w433]
        # "Histogram of angles (this method is abandoned)"
        n212 = call <vilib>:"Histogram.vi"("X"=w433) -> ()  [unwired: 7 in, 4 out]
        n213 = call <vilib>:"Std Deviation and Variance.vi"("X"=w433) -> ("mean"=w434:dbl, "standard deviation"=w435:dbl)  [unwired: 1 in, 1 out]
      }
    }
    frame Enabled {
    }
  }
  n214 = disable-structure shown="Disabled" {
    disable-tunnel: w45 -> [w450 _]
    disable-tunnel: w30 -> [w447 _]
    frame Disabled {
      n215 = in-place {
        in-place-border: w450 -> [w454]
        in-place-border: [w451] -> w449
        in-place-border: w447 -> [w452]
        in-place-border: [w453] -> w444
        w458 = u16 0 items=["Y", "X", "X and Y"] ("range type")
        # "Exclude poor fits"
        n216 = call <vilib>:"Std Deviation and Variance.vi"("X"=w452) -> ("mean"=w456:dbl, "standard deviation"=w462:dbl)  [unwired: 1 in, 1 out]
        n217 = Multiply(x=w462, y="Keep N Devs") -> (x*y=w461:dbl)
        n218 = Add(x=w456, y=w461) -> (x+y=w460:dbl)
        n219 = Subtract(x=w456, y=w461) -> (x-y=w459:dbl)
        n220 = Build Array(w460, w459) -> (w457:dbl[])
        n221 = call-poly <vilib>:"Remove Outliers.vi"("Y"=w452, "X"=w454, "range type"=w458, "Range"=w457) -> ("Y Out"=w453:dbl[], "X Out"=w451:dbl[])  [unwired: 7 in, 3 out]
      }
      "Slope Error" <- w444
      n222 = Negate(x=w449) -> (-x=w448:dbl[])
      "Fit Slopes" <- w448
      n223 = in-place {
        in-place-border: w448 -> [w482]
        in-place-border: w444 -> [w475]
        in-place-border: [w478] -> w446
        in-place-border: [w474] -> w445
        w484 = T3 0 items=["Least Square", "Least Absolute Residual", "Bisquare"] ("method")
        # "Weighted mean of slopes"
        n224 = Array Size(array=w475) -> (size(s)=→"Num slope errors":i32)
        n225 = Array Size(array=w482) -> (size(s)=w486:i32)
        "Num slopes" <- w486
        n226 = for {
          N: w486 -> [_]
          tunnel: [w487] -> w485 mode=indexing
          i -> [w487]
        }
        n227 = Reciprocal(x=w475) -> (1/x=w480:dbl[])
        n228 = To Double Precision Float(number=w485) -> (double precision float=w481:dbl[])
        n229 = call <vilib>:"Linear Fit.vi"("Y"=w482, "X"=w481, "Weight"=w480, "tolerance"=0.0001, "method"=w484) -> ("slope"=w479:dbl, "intercept"=w478:dbl)  [unwired: 6 in, 3 out]
        "Slope" <- w478
        n230 = call-poly <vilib>:"Linear Fit Intervals.vi"("Y"=w482, "confidence level"=0.68, "X"=w481, "Weight"=w480, "slope"=w479, "intercept"=w478) -> ("delta intercept"=w474:dbl)  [unwired: 5 in, 4 out]
        "Error (Slope)" <- w474
      }
      n231 = in-place {
        in-place-border: w446 -> [w466]
        in-place-border: [w464] -> _
        in-place-border: w445 -> [w465]
        in-place-border: [w463] -> _
        (unwired) 0.026
        # "Skew angle calculation (this method is abandoned)"
        n232 = Inverse Tangent(1:w466) -> (0:w464:dbl)
        "Radians" <- w464
        n233 = in-place {
          in-place-border: w464 -> [w472]
          in-place-border: w465 -> [w468]
          in-place-border: [w467] -> w463
          w473 = 1.0
          # "[1/(1+theta^2)]dtheta"
          n234 = Square(x=w472) -> (x^2=w471:dbl)
          n235 = Add(x=w473, y=w471) -> (x+y=w470:dbl)
          n236 = Divide(x=w473, y=w470) -> (x/y=w469:dbl)
          n237 = Multiply(x=w469, y=w468) -> (x*y=w467:dbl)
          "Error (Radians)" <- w467
        }
      }
    }
    frame Enabled {
    }
  }
